vi "Upgrade Component Dependencies.vi"(0 "NI Build Specification_LV In":refnum<class "NI Build Specification_LV.lvclass">, 11 "error in (no error)":errorcluster) -> (4 "NI Build Specification_LV Out":refnum<class "NI Build Specification_LV.lvclass">, 15 "error out":errorcluster)   [LabVIEW 2017, in "CL_G3_VIComponentBuilder.lvlib" / "NI Build Specification_LV.lvclass"]
doc: "Upgrades a component's dependencies. For example, in the case of a VI Package, this VI edits the VIPB to use the latet version of a VI Package's dependencies."
uses:
  NI Build Specification_LV.lvclass
  Exports/Export.lvclass
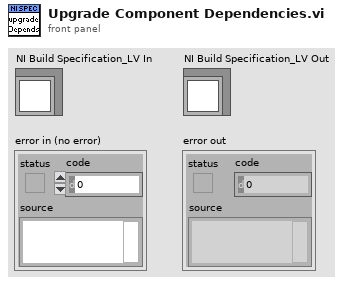
[diagram p1: front panel]
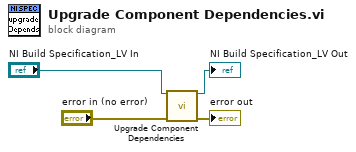
[diagram p0: block diagram]
diagram:
  n1 = call-parent "Upgrade Component Dependencies.vi"("Export In"="NI Build Specification_LV In", "error in (no error)"="error in (no error)") -> ("Export Out"=→"NI Build Specification_LV Out":refnum<class "NI Build Specification_LV.lvclass">, "error out"=→"error out":errorcluster)  [unwired: 12 in]
